vi "Read SPI Response for SPI Transactions 128-bit.vi"(8 "error in":errorcluster, 9 "Read Data? (T)":bool=TRUE, 11 "SPI Engine Resources":T3={"To SPI Engine Data FIFO"="DLU To SPI Engine Data FIFO", "From SPI Engine Data FIFO"="SPI Engine to DLU Data FIFO", "Data to SPI Engine Cache Register"="Data to SPI Engine (Cache)", "SPI Transaction Settings Cache Register"="SPI PHY Settings to SPI Engine (Cache)"}) -> (0 "error out":errorcluster, 1 "Read Data Valid?":bool, 2 "Read Data":T1, 3 "SPI Engine Resources":T3={"To SPI Engine Data FIFO"="DLU To SPI Engine Data FIFO", "From SPI Engine Data FIFO"="SPI Engine to DLU Data FIFO", "Data to SPI Engine Cache Register"="Data to SPI Engine (Cache)", "SPI Transaction Settings Cache Register"="SPI PHY Settings to SPI Engine (Cache)"})   [LabVIEW 2015, in "SPI API.lvlib"]
doc: "This VI reads data transfers data from SPI Engine if valid data is available. If the Read Data Valid? output is not true, then the data output from this VI is invalid. Set the Read Data? control to false to skip reading.\n\n<b> Note: It is recommended to read the \"Read Data Valid\" output to check if SPI Engine consumed the data written, if not data has to be re-read. </b>"
uses:
  SPI API.lvlib
  Controls/SPI Engine Resources 128-bit.ctl
  Controls/SPI API Response Data 128-bit.ctl
  Controls/SPI API Data 128-bit.ctl
  <vilib>/rvi/DataTransferAndStorage/Container/Common/niFpgaContainerExecOnDevCompGetState.vi
  <vilib>/rvi/Emulation/niFpgaEmulationIsFPGAContextNoSignature.vi
  <vilib>/rvi/Emulation/niFpgaSctlEmulationGetInTimedLoop.vi
  <vilib>/rvi/errors/niFpgaSetErrorForExecOnDevCompSimple.vi
  <vilib>/rvi/eio/common/nirviEmuReportErrorAndStop.vi
  <vilib>/rvi/DataTransferAndStorage/Container/Common/niFpgaContainerGetUniqueNameForEmu.vi
  <vilib>/rvi/FIFO/Fifo_Resource/nirvififoEmulationSetSize.vi
  <vilib>/rvi/FIFO/Fifo_Resource/nirviFifoEmulationQueueMgr.vi
  <instcachedir>/0/nirviFifoEmulationQueueMgr_E5CAEC123FF24DC58D834DCA3CDAA9B5.lvgen/nirviFifoEmulationQueueMgr_E5CAEC123FF24DC58D834DCA3CDAA9B5_013.vi
  <vilib>/rvi/FIFO/Fifo_Resource/nirvififoEmulationDetermineInputValidOut.vi
  <vilib>/rvi/FIFO/Fifo_Resource/nirvififoEmulationCreateLock.vi
  <vilib>/rvi/Emulation/niFpgaProcessEmulError.vi
  <vilib>/rvi/FIFO/Fifo_Resource/nirvififoEmulationObtainLock.vi
  <vilib>/rvi/FIFO/Fifo_Resource/nirvififoEmulationReleaseLock.vi
  <vilib>/rvi/occurrence/nirviWaitOnOccurrenceBase.vi
  <vilib>/rvi/errors/nirviReportUnexpectedCaseInternalError.vi
  <vilib>/rvi/errors/nirviReportUnexpectedCaseInternalError (U32).vi
  <vilib>/Utility/error.llb/Clear Errors.vi
  <vilib>/rvi/interface/RandomDataEmulation/niFpgaRandomDataHandleErrors.vi
  <vilib>/rvi/DataTransferAndStorage/Container/XNode/niFpgaContainer.xnode
  <vilib>/rvi/FIFO/Fifo_Resource/niFpgaFifoEmulationRefIn.vi
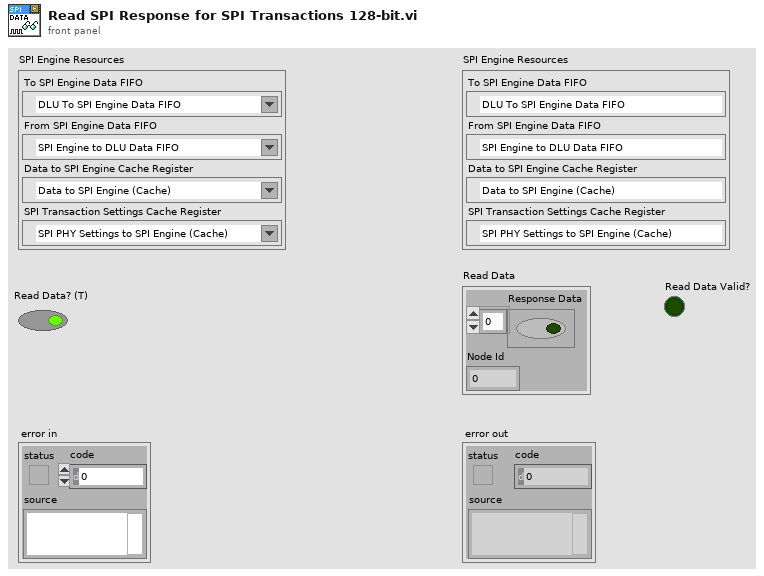
[diagram p1: front panel]
types:
  T1 = typedef "SPI API.lvlib/SPI API Response Data 128-bit.ctl" = cluster{"Response Data":T2, "Node Id":u16}
  T2 = typedef "SPI API.lvlib/SPI API Data 128-bit.ctl" = bool[]
  T3 = typedef "SPI API.lvlib/SPI Engine Resources 128-bit.ctl" = cluster{"To SPI Engine Data FIFO":refnum<k21>, "From SPI Engine Data FIFO":refnum<k21>, "Data to SPI Engine Cache Register":refnum<k21>, "SPI Transaction Settings Cache Register":refnum<k21>}
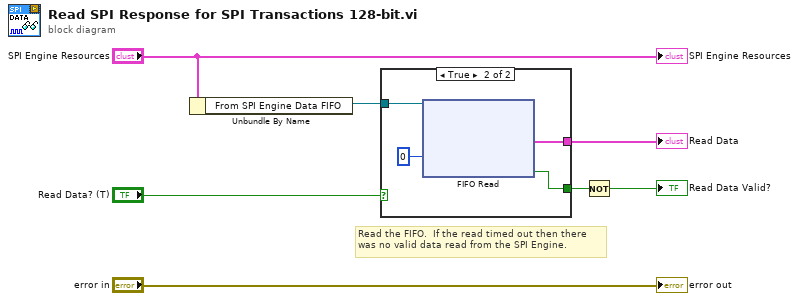
[diagram p0: block diagram]
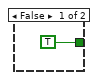
[diagram p2: hidden frame]
diagram:
  # "Read the FIFO.  If the read timed out then there\nwas no valid data read from the SPI Engine."
  n1 = Unbundle By Name("SPI Engine Resources") -> ("From SPI Engine Data FIFO"=w5:refnum<k21>)
  n2 = case shown="True" "Read Data? (T)" {
    tunnel: w5 -> [_ w12]
    tunnel: [TRUE ("Timed Out?") w11] -> w4
    tunnel: [_ w10] -> w1
    frame False {
    }
    frame True {
      n3 = xnode ("FIFO Read")("Timeout"=0, "FIFO In"=w12) -> ("Element"=w10:cluster{"Data to Node":bool[], "Node Id":u16}, "Timed Out?"=w11:bool)  [unwired: 1 out]
    }
  }
  "Read Data" <- w1
  n4 = Not(x=w4) -> (.not. x?=→"Read Data Valid?":bool)
  "error out" <- "error in"
  "SPI Engine Resources" <- "SPI Engine Resources"
